vi "Show UI.vi"(8 "error in (no error)":errorcluster, 11 "Actor wUI in":refnum<class "Actor wUI.lvclass">) -> (0 "error out":errorcluster, 3 "Actor wUI out":refnum<class "Actor wUI.lvclass">)   [LabVIEW 2017, in "Framework.lvlib" / "Actor wUI.lvclass"]
uses:
  Actor wUI.lvclass
  Actor wUI.lvclass/Actor wUI.ctl
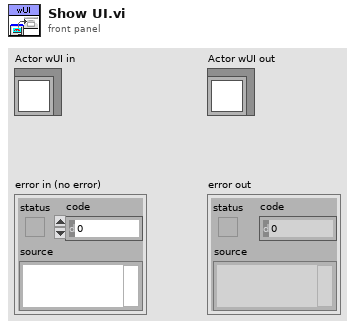
[diagram p1: front panel]
types:
  T1 = enum32{"Invalid", "Standard", "Closed", "Hidden", "Minimized", "Maximized"}
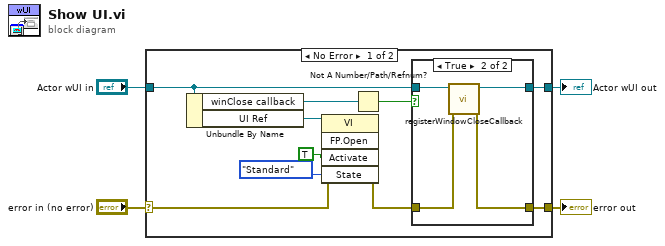
[diagram p0: block diagram]
diagram:
  n1 = case shown="No Error" "error in (no error)" {
    selector: "error in (no error)" -> [w11 w22]
    tunnel: [w6 w22] -> w3
    tunnel: [w8 w21] -> w1
    tunnel: "Actor wUI in" -> [w9 w21]
    frame No Error {
      n2 = Unbundle By Name(w9) -> ("winClose callback"=w10:refnum<k27>, "UI Ref"=w14:refnum<vi>)
      n3 = invoke class="VI" method="FP.Open"(reference=w14, error in=w11, "Activate"=TRUE ("Activate?"), "State"=T1."Standard") -> (error out=w7:errorcluster)  [unwired: 1 in, 4 out]
      n4 = Not A Number/Path/Refnum?(number/path/refnum=w10) -> (NaN/Path/Refnum?=w5:bool)
      n5 = case shown="True" w5 {
        tunnel: w9 -> [w16 w20]
        tunnel: [w16 w19] -> w8
        tunnel: w7 -> [w15 w18]
        tunnel: [w15 w17] -> w6
        frame False {
        }
        frame True {
          n6 = call "registerWindowCloseCallback.vi"("error in (no error)"=w18, "Actor wUI in"=w20) -> ("error out"=w17:errorcluster, "Actor wUI out"=w19:refnum<class "Actor wUI.lvclass">)  [unwired: 8 in]
        }
      }
    }
    frame Error {
    }
  }
  "error out" <- w3
  "Actor wUI out" <- w1
